vi "Create User.vi"(8 "error in (no error)":errorcluster caption="错误输入（无错误）", 11 "SQL Factory 输入":refnum<class "SQL Factory.lvclass">) -> (0 "error out":errorcluster caption="错误输出", 2 "Abstract User.lvclass":refnum<class "Abstract User.lvclass">, 3 "SQL Factory 输出":refnum<class "SQL Factory.lvclass">)   [LabVIEW 2017, in "SQL Factory.lvclass"]
uses:
  SQL Factory.lvclass
  Abstract User/Abstract User.lvclass
  SQL User/SQL User.lvclass
  Abstract Factory/Abstract Factory.lvclass
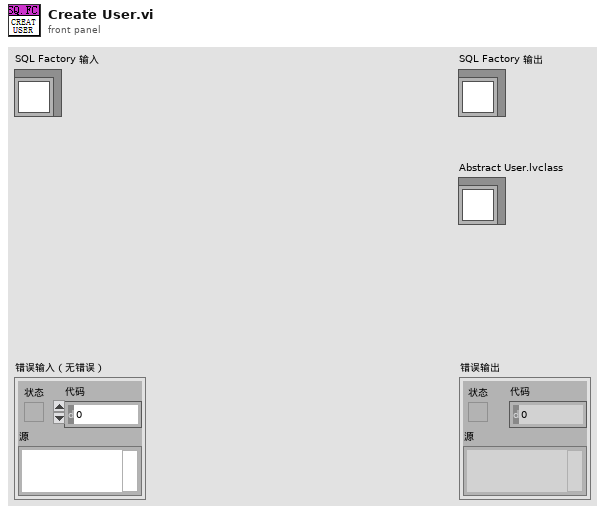
[diagram p1: front panel]
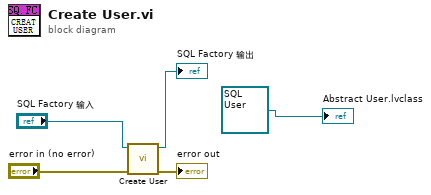
[diagram p0: block diagram]
diagram:
  n1 = call-parent "Create User.vi"("error in (no error)"="error in (no error)", "Abstract Factory 输入"="SQL Factory 输入") -> ("error out"=→"error out":errorcluster, "Abstract Factory 输出"=→"SQL Factory 输出":refnum<class "SQL Factory.lvclass">)  [unwired: 7 in, 1 out]
  "Abstract User.lvclass" <- refnum<class "SQL User.lvclass"> refnum ("SQL User.lvclass")
